vi "CRio9063_4chan_9222.vi"() -> ()   [LabVIEW 2014]
uses:
  <vilib>/rvi/eio/nirviErrorMerge/nirviErrorMerge.xnode
  <vilib>/rvi/eio/common/nirviEmuClasses.ctl
  <vilib>/rvi/eio/common/nirviEmuTemplateMethod_errors.vi
  <vilib>/rvi/eio/nirviEIOMethodImplementation/nirviEIOMethodImplementation.xnode
  <vilib>/eio/EIOGrowableMethodNode/genericMethod/EIOGrowableMethodNode.xnode
  <vilib>/rvi/DataTransferAndStorage/Container/XNode/niFpgaContainer.xnode
  <vilib>/eio/EIONode/EIONode.xnode
  <vilib>/rvi/interface/RandomDataEmulation/nirviRandomDataFpgaReadWriteTemplate.vi
panel:
  in  "User Fpga Led":bool
  out "Chassis Temperature":i16
  in  "System Reset":bool
  in  "Sample Period (uSec)":u32=2
  out "Timed Out":bool
  out "Overwrite":bool
  out "Sample Gated":bool
  in  "USER FPGA LED":bool
  in  "Boolean":bool
  out "Stopped":bool
  out "nChannels":i32=8
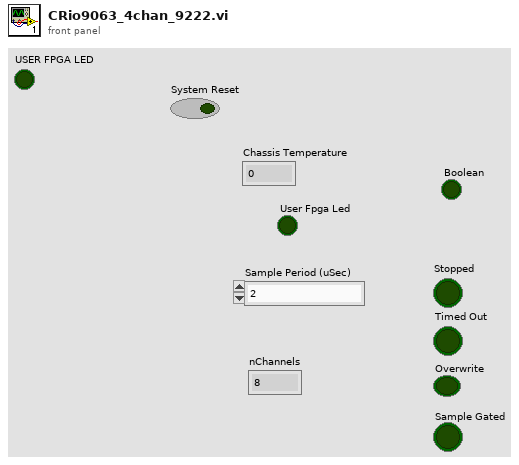
[diagram p1: front panel]
types:
  T1 = typedef "nirviEmuClasses.ctl" = enum16{"IO Read", "IO Write", "Method", "Property Read", "Property Write"}
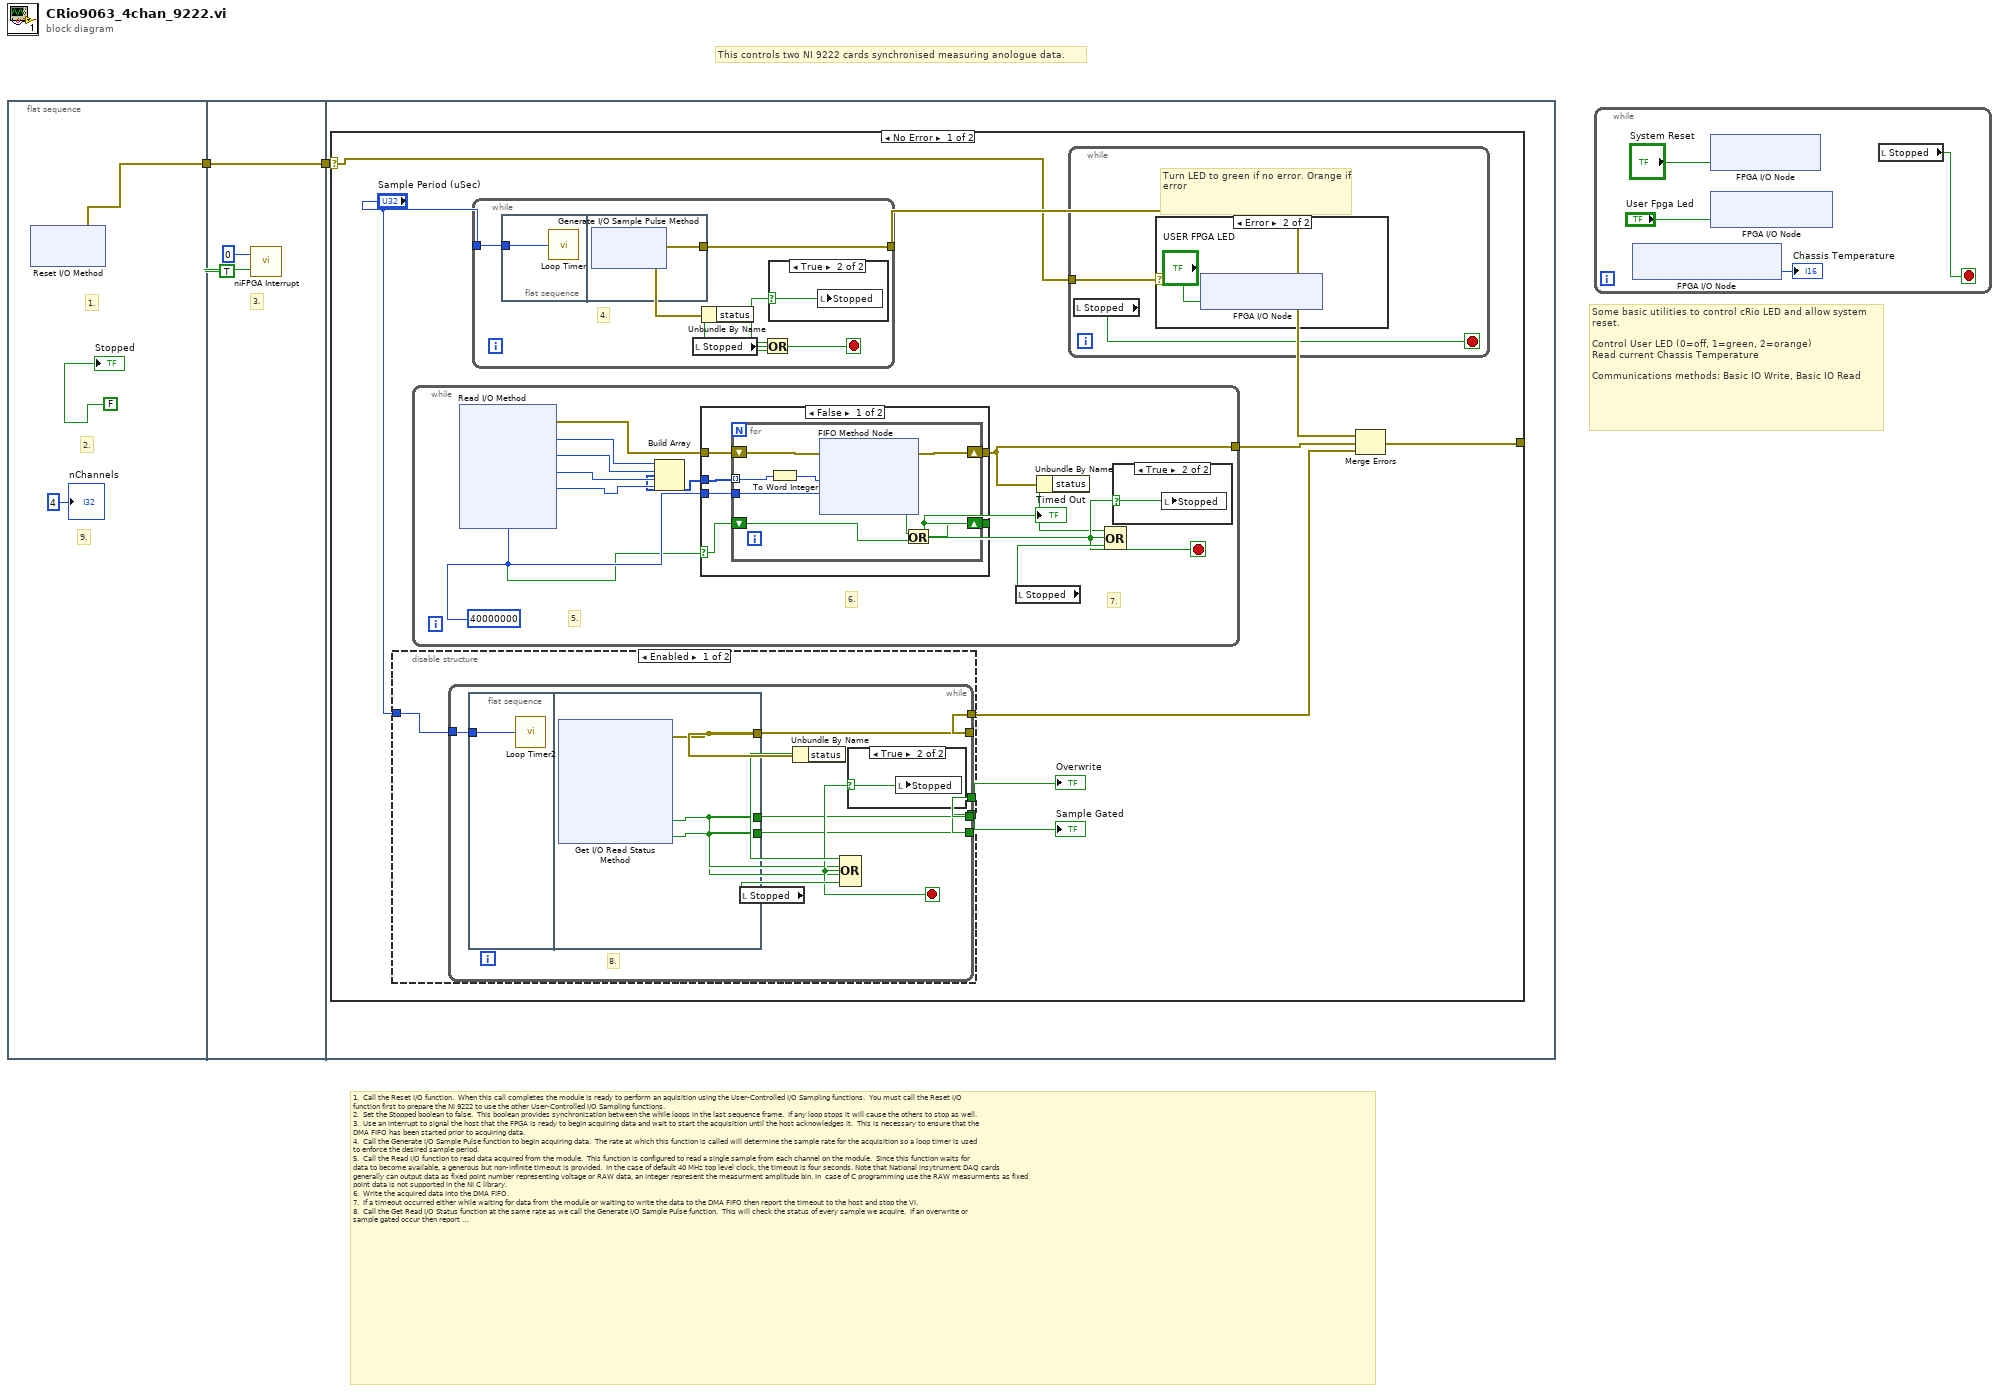
[diagram p0: block diagram]
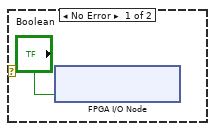
[diagram p2: hidden frame]
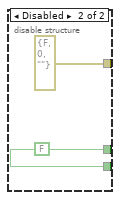
[diagram p4: hidden frame]
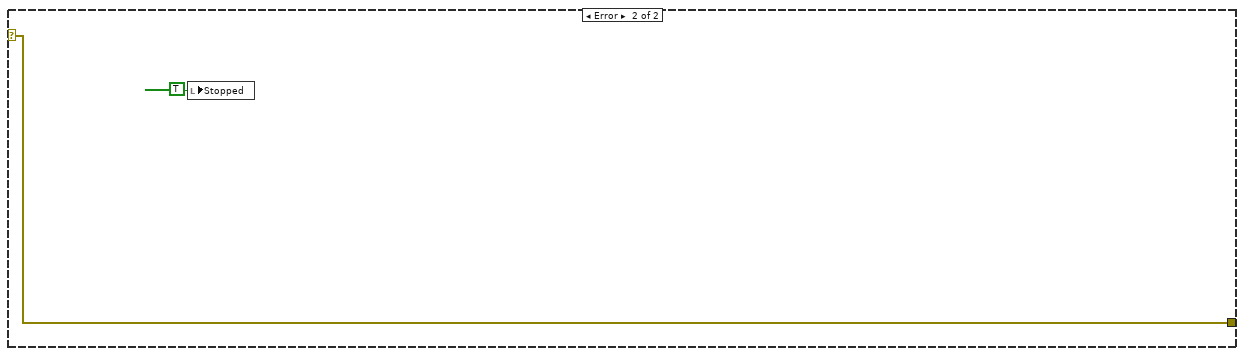
[diagram p8: hidden frame]
diagram:
  # "Some basic utilities to control cRio LED and allow system reset. \n\nControl User LED (0=off, 1=green, 2=orange)\nRead current Chassis Temperature\n\nCommunications methods: Basic IO Write, Basic IO Read"
  # "This controls two NI 9222 cards synchronised measuring anologue data."
  # "1.  Call the Reset I/O function.  When this call completes the module is ready to perform an aquisition using the User-Controlled I/O Sampling functions.  You must call the Reset I/O \nfunction first to prepare the NI 9222 to use the other User-Controlled I/O Sampling functions.\n2.  Set the Stopped boolean to false.  This boolean provides synchronization between the while loops in the last sequence frame.  If any loop stops it will cause the others to stop as well.\n3.  Use an interrupt to signal the host that the FPGA is ready to begin acquiring data and wait to start the acquisition until the host acknowledges it.  This is necessary to ensure that the \nDMA FIFO has been started prior to acquiring data.\n4.  Call the Generate I/O Sample Pulse function to begin acquiring data.  The rate at which this function is called will determine the sample rate for the acquisition so a loop timer is used\nto enforce the desired sample period.\n5.  Call the Read I/O function to read data acquired from the module.  This function is configured to read a single sample from each channel on the module.  Since this function waits for\ndata to become available, a generous but non-infinite timeout is provided.  In the case of default 40 MHz top level clock, the timeout is four seconds. Note that National insytrument DAQ cards \ngenerally can output data as fixed point number representing voltage or RAW data, an integer represent the measurment amplitude bin. In  case of C programming use the RAW measurments as fixed \npoint data is not supported in the NI C library. \n6.  Write the acquired data into the DMA FIFO.\n7.  If a timeout occurred either while waiting for data from the module or waiting to write the data to the DMA FIFO then report the timeout to the host and stop the VI.\n8.  Call the Get Read I/O Status function at the same rate as we call the Generate I/O Sample Pulse function.  This will check the status of every sample we acquire.  If an overwrite or \nsample gated occur then report the status to the host and stop the VI.  This loop is encased in a diagram disable struction to make it easily removable from the application.  Calling the \nGet Read I/O Status function is useful for development and debugging but not strictly necessary for deployment if there is no variable timing in the application.  In the above example, it\nis not possible to get a sample gated status unless the top loop's sample period is less than the minimum sample period supported by the module.  However, this application could \nproduce an overwrite status if the host VI cannot read from the DMA FIFO fast enough.\n9. I constant indicating the number of channels the FPGA is recording from. This is manually set."
  n1 = flat-sequence {
    tunnel: [w4] -> w2
    tunnel: w2 -> [w50]
    tunnel: [w50] -> w1
    tunnel: w1 -> [w53]
    frame #0 {
      # "9."
      # "2."
      # "1."
      n2 = xnode "Reset I/O Method"() -> ("error out"=w4:errorcluster)  [unwired: 2 in, 1 out]
      "Stopped" <- FALSE ("Stopped")
      "nChannels" <- 4
    }
    frame #1 {
      # "3."
      n3 = call <vilib>:"niFPGA Interrupt.vi"("Wait Until Cleared (F)"=TRUE ("Wait Until Cleared"), "IRQ Number (0)"=u8 0 ("IRQ Number")) -> ()  [unwired: 1 in]
    }
    frame #2 {
      n4 = case shown="No Error" w53 {
        selector: w53 -> [w54 w514]
        tunnel: [w58 w514] -> _
        frame No Error {
          n5 = disable-structure shown="Enabled" {
            disable-tunnel: [w69 errorcluster {"status"=FALSE, "code"=0, "source"=""} ("error out")] -> w59
            disable-tunnel: "Sample Period (uSec)" -> [w68 _]
            disable-tunnel: [w67 w250] -> w55
            disable-tunnel: [w66 w250] -> w56
            frame Enabled {
              n6 = while {
                tunnel: [w76] -> w69
                tunnel: w68 -> [w75]
                tunnel: [w71] -> w67
                tunnel: [w70] -> w66
                stop <- w72 stop-if-true
                # "8."
                n7 = flat-sequence {
                  tunnel: w75 -> [w78]
                  tunnel: [w81] -> w76
                  tunnel: [w80] -> w71
                  tunnel: [w79] -> w70
                  frame #0 {
                    n8 = call "Loop Timer2"("Count(uSec)"=w78) -> ()  [unwired: 1 out]
                  }
                  frame #1 {
                    n9 = xnode "Get I/O Read Status Method"() -> ("error out"=w81:errorcluster, "Overwrite"=w80:bool, "Sample Gated"=w79:bool)  [unwired: 5 in, 4 out]
                  }
                }
                n10 = local read "Stopped"() -> (w74:bool)
                n11 = Unbundle By Name(w76) -> ("status"=w73:bool)
                n12 = Compound Arithmetic op=OR(w73, w71, w70, w74) -> (w72:bool)
                n13 = case shown="True" w72 {
                  selector: w72 -> [_ w77]
                  frame False {
                  }
                  frame True {
                    n14 = local write "Stopped"(w77) -> ()
                  }
                }
              }
            }
            frame Disabled {
              w250 = FALSE ("Overwrite")
            }
          }
          "Overwrite" <- w55
          "Sample Gated" <- w56
          n15 = while {
            tunnel: [w262] -> w60
            stop <- w253 stop-if-true
            w263 = 40000000 ("Timeout")
            # "7."
            # "6."
            # "5."
            n16 = xnode ("Read I/O Method")("Timeout"=w263) -> ("error out"=w261:errorcluster, "Mod1/AI0"=w255:i16, "Mod1/AI1"=w264:i16, "Mod1/AI2"=w257:i16, "Mod1/AI3"=w256:i16, "Timed Out"=w260:bool)  [unwired: 5 in, 4 out]
            n17 = Build Array(w255, w264, w257, w256) -> (w254:i16[])
            n18 = case shown="False" w260 {
              selector: w260 -> [w267 w280]
              tunnel: w263 -> [w271 _]
              tunnel: [w270 w281] -> w262
              tunnel: [w269 w280] -> w258
              tunnel: w261 -> [w268 w281]
              tunnel: w254 -> [w266 _]
              frame False {
                n19 = for {
                  tunnel: w266 -> [w275] mode=indexing
                  shift-right: [w278] -> w270
                  shift-left: w268 -> [w279]
                  tunnel: w271 -> [w273]
                  shift-right: [w277] -> w269
                  shift-left: w267 -> [w276]
                  n20 = To Word Integer(number=w275) -> (16bit integer=w274:i16)
                  n21 = xnode ("FIFO Method Node")("Element"=w274, "Timeout"=w273, "error in (no error)"=w279) -> ("Timed Out?"=w272:bool, "error out"=w278:errorcluster)  [unwired: 1 in, 1 out]
                  n22 = Or(x=w272, y=w276) -> (x .or. y?=w277:bool)
                }
              }
              frame True {
              }
            }
            "Timed Out" <- w258
            n23 = local read "Stopped"() -> (w259:bool)
            n24 = Unbundle By Name(w262) -> ("status"=w252:bool)
            n25 = Compound Arithmetic op=OR(w252, w258, w259) -> (w253:bool)
            n26 = case shown="True" w253 {
              selector: w253 -> [_ w265]
              frame False {
              }
              frame True {
                n27 = local write "Stopped"(w265) -> ()
              }
            }
          }
          n28 = while {
            tunnel: "Sample Period (uSec)" -> [w466]
            tunnel: [w463] -> w61
            stop <- w462 stop-if-true
            # "4."
            n29 = flat-sequence {
              tunnel: w466 -> [w468]
              tunnel: [w469] -> w463
              frame #0 {
                n30 = call "Loop Timer"("Count(uSec)"=w468) -> ()  [unwired: 1 out]
              }
              frame #1 {
                n31 = xnode "Generate I/O Sample Pulse Method"() -> ("error out"=w469:errorcluster)  [unwired: 2 in, 1 out]
              }
            }
            n32 = local read "Stopped"() -> (w465:bool)
            n33 = Unbundle By Name(w463) -> ("status"=w464:bool)
            n34 = Or(x=w464, y=w465) -> (x .or. y?=w462:bool)
            n35 = case shown="True" w462 {
              selector: w462 -> [_ w467]
              frame False {
              }
              frame True {
                n36 = local write "Stopped"(w467) -> ()
              }
            }
          }
          n37 = while {
            tunnel: w54 -> [w63]
            stop <- w62 stop-if-true
            # "Turn LED to green if no error. Orange if error"
            n38 = local read "Stopped"() -> (w62:bool)
            n39 = case shown="Error" w63 {
              frame No Error {
                n40 = xnode "FPGA I/O Node"("USER FPGA LED"="Boolean") -> ()  [unwired: 1 in, 1 out]
              }
              frame Error {
                n41 = xnode "FPGA I/O Node"("USER FPGA LED"="USER FPGA LED") -> ()  [unwired: 1 in, 1 out]
              }
            }
          }
          n42 = Merge Errors(w61, w60, w59) -> (w58:errorcluster)
        }
        frame Error {
          n43 = local write "Stopped"(TRUE ("Stopped")) -> ()
        }
      }
    }
  }
  n44 = while {
    stop <- w516 stop-if-true
    n45 = xnode "FPGA I/O Node"() -> ("Chassis Temperature"=→"Chassis Temperature":i16)  [unwired: 1 in, 1 out]
    n46 = xnode "FPGA I/O Node"("System Reset"="System Reset") -> ()  [unwired: 1 in, 1 out]
    n47 = xnode "FPGA I/O Node"("USER FPGA LED"="User Fpga Led") -> ()  [unwired: 1 in, 1 out]
    n48 = local read "Stopped"() -> (w516:bool)
  }
